vi "Fmin,Fmax to CF,BW.vi"(8 "Fmax":dbl, 10 "Fmin":dbl) -> (0 "BW":dbl, 2 "CF":dbl)   [LabVIEW 2020]
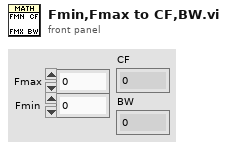
[diagram p1: front panel]
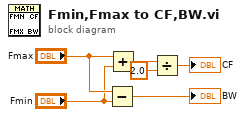
[diagram p0: block diagram]
diagram:
  n1 = Subtract(x="Fmax", y="Fmin") -> (x-y=→"BW":dbl)
  n2 = Add(x="Fmax", y="Fmin") -> (x+y=w5:dbl)
  n3 = Divide(x=w5, y=2.0) -> (x/y=→"CF":dbl)
